vi "SendHardwareErrorStatus.vi"(8 "error in (no error)":errorcluster, 9 "EDP Hardware Labview Error Status":T1, 11 "Handle In":u32 format="%x") -> (0 "error out":errorcluster, 3 "Handle Out":u32 format="%x")   [LabVIEW 2020]
uses:
  <userlib>/Beckhoff-LabVIEW-Interface/_DependsOn/With TypeResolving/Write Sync Single TypeResolved.vi
panel:
  out "Has Matched? 3":bool
  out "Write Status 3":bool
  in  "WriteGrpSymbols 2":string[](array[string])=["192.168.0.20.1.1:851::GVL_LabviewDataShare.in_bAardvarkBoardError_labview", "192.168.0.20.1.1:851::GVL_LabviewDataShare.in_bAsic1CalibrationCompleted_labview", "192.168.0.20.1.1:851::GVL_LabviewDataShare.in_bAsic1CalibrationInProgress_labview", "192.168.0.20.1.1:851::GVL_LabviewDataShare.in_bAsic1CalibrationSuccess_labview", "192.168.0.20.1.1:851::GVL_LabviewDataShare.in_bAsic1FFTCompleted_labview", "192.168.0.20.1.1:851::GVL_LabviewDataShare.in_bAsic1FFTInProgress_labview", "192.168.0.20.1.1:851::GVL_LabviewDataShare.in_bAsic1FFTSuccess_labview", "192.168.0.20.1.1:851::GVL_LabviewDataShare.in_bAsic2CalibrationCompleted_labview", "192.168.0.20.1.1:851::GVL_LabviewDataShare.in_bAsic2CalibrationInProgress_labview", "192.168.0.20.1.1:851::GVL_LabviewDataShare.in_bAsic2CalibrationSuccess_labview", "192.168.0.20.1.1:851::GVL_LabviewDataShare.in_bAsic2FFTCompleted_labview", "192.168.0.20.1.1:851::GVL_LabviewDataShare.in_bAsic2FFTInProgress_labview", "192.168.0.20.1.1:851::GVL_LabviewDataShare.in_bAsic2FFTSuccess_labview", "192.168.0.20.1.1:851::GVL_LabviewDataShare.in_bCalResultsDBStoreSuccess_labview", "192.168.0.20.1.1:851::GVL_LabviewDataShare.in_bFFTResultsDBStoreSuccess_labview", "192.168.0.20.1.1:851::GVL_LabviewDataShare.in_bLabviewHandshakeBit", "192.168.0.20.1.1:851::GVL_LabviewDataShare.in_bLabviewResetComplete_labview", "192.168.0.20.1.1:851::GVL_LabviewDataShare.in_bLabviewResetSuccess_labview", "192.168.0.20.1.1:851::GVL_LabviewDataShare.in_bNIDaqError_labview", "192.168.0.20.1.1:851::GVL_LabviewDataShare.in_bPTC04BoardError_labview", "192.168.0.20.1.1:851::GVL_LabviewDataShare.in_bStartupInitializationCompleted_labview", "192.168.0.20.1.1:851::GVL_LabviewDataShare.in_bStartupInitializationSuccess_labview", "192.168.0.20.1.1:851::GVL_LabviewDataShare.in_strAsic1SerialNo_labview", "192.168.0.20.1.1:851::GVL_LabviewDataShare.in_strAsic2SerialNo_labview"]
  out "Write Status 2":bool
  out "Has Matched? 2":bool
  out "Write Status":bool
  out "Has Matched?":bool
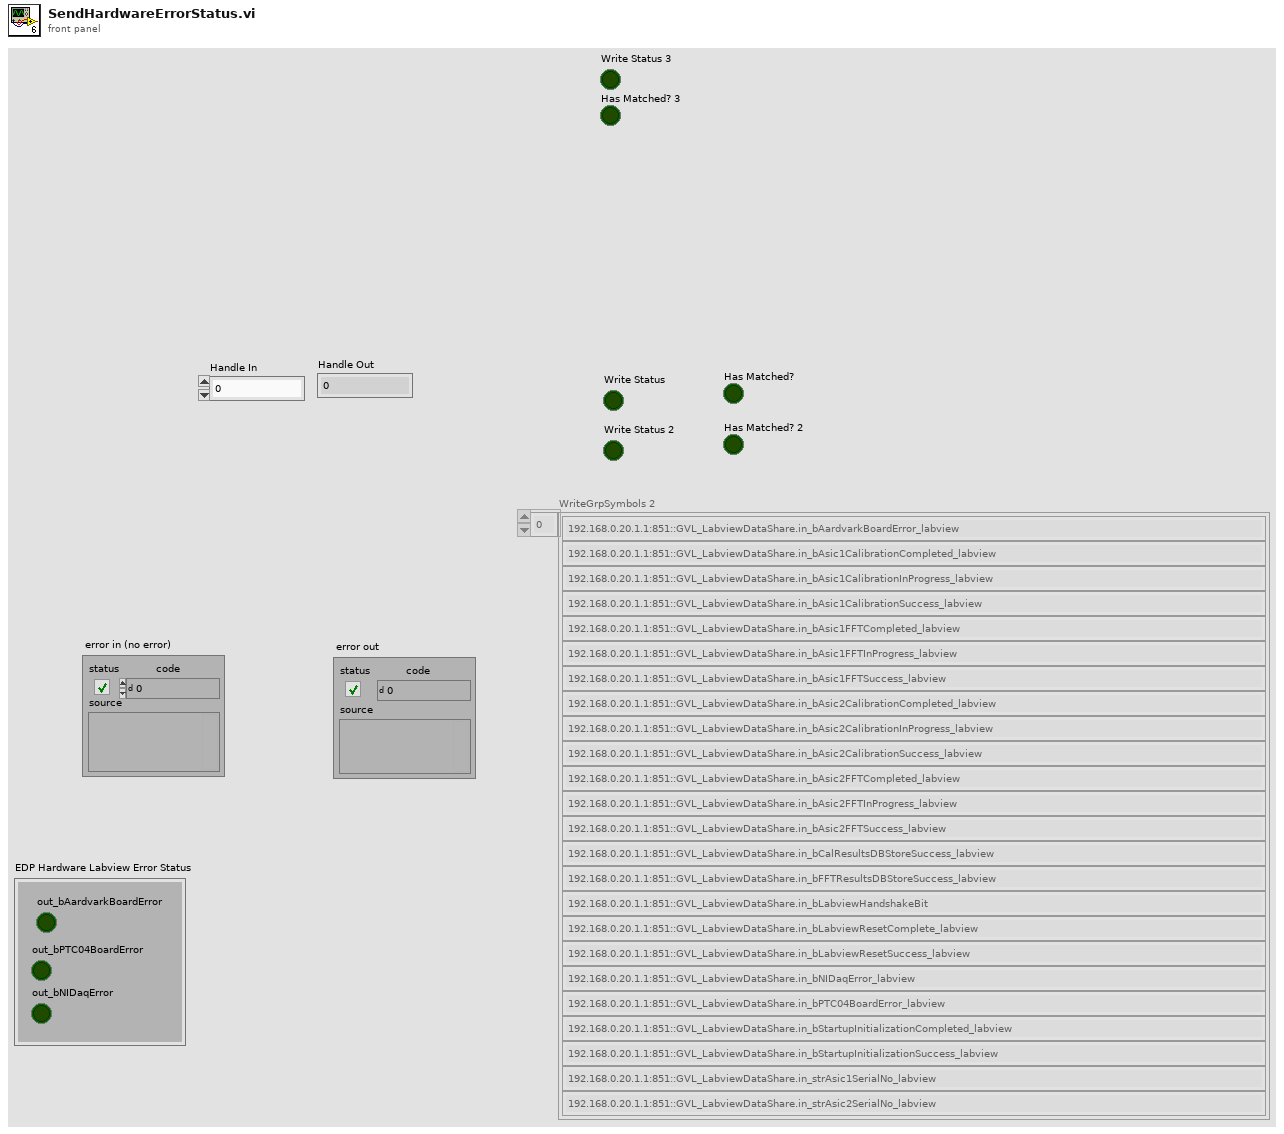
[diagram p1: front panel]
types:
  T1 = cluster{"out_bAardvarkBoardError":bool, "out_bPTC04BoardError":bool, "out_bNIDaqError":bool}
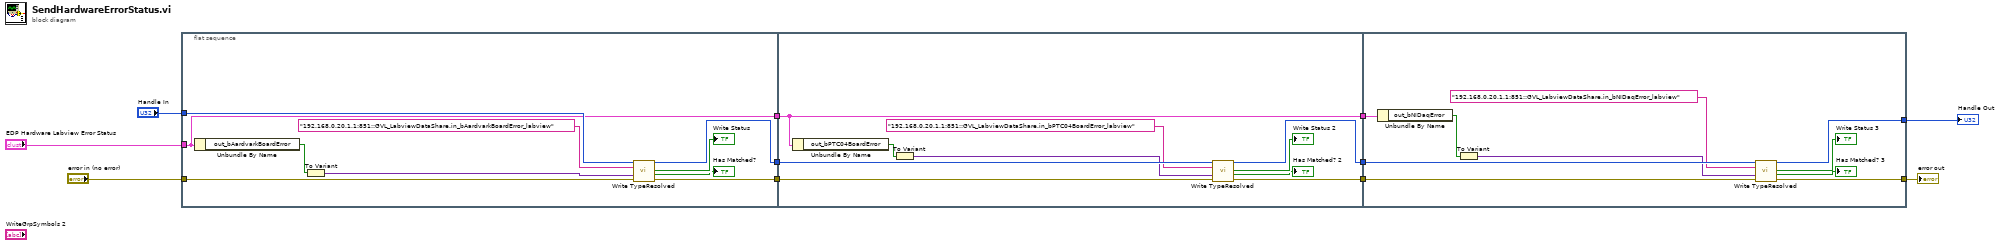
[diagram p0: block diagram]
diagram:
  n1 = flat-sequence {
    tunnel: "Handle In" -> [w21]
    tunnel: [w20] -> w11
    tunnel: [w19] -> w10
    tunnel: "error in (no error)" -> [w18]
    tunnel: "EDP Hardware Labview Error Status" -> [w15]
    tunnel: [w15] -> w9
    tunnel: w11 -> [w31]
    tunnel: w10 -> [w30]
    tunnel: w9 -> [w22]
    tunnel: [w24] -> w3
    tunnel: [w23] -> w2
    tunnel: [w22] -> w1
    tunnel: [w36] -> w5
    tunnel: [w38] -> w6
    tunnel: w3 -> [w39]
    tunnel: w2 -> [w37]
    tunnel: w1 -> [w41]
    frame #0 {
      n2 = Unbundle By Name(w15) -> ("out_bAardvarkBoardError"=w17:bool)
      n3 = To Variant(anything=w17) -> (Variant=w16:variant)
      n4 = call-poly <userlib>:"Write TypeResolved.vi"("Handle"=w21, "SymbolName"="192.168.0.20.1.1:851::GVL_LabviewDataShare.in_bAardvarkBoardError_labview", "WData"=w16, "error constant"=w18) -> ("Handle"=w20:u32, "Write Status?"=→"Write Status":bool, "Has Matched?"=→"Has Matched?":bool, "error out"=w19:errorcluster)  [unwired: 8 in]
    }
    frame #1 {
      n5 = Unbundle By Name(w22) -> ("out_bPTC04BoardError"=w29:bool)
      n6 = To Variant(anything=w29) -> (Variant=w28:variant)
      n7 = call-poly <userlib>:"Write TypeResolved.vi"("Handle"=w31, "SymbolName"="192.168.0.20.1.1:851::GVL_LabviewDataShare.in_bPTC04BoardError_labview", "WData"=w28, "error constant"=w30) -> ("Handle"=w23:u32, "Write Status?"=→"Write Status 2":bool, "Has Matched?"=→"Has Matched? 2":bool, "error out"=w24:errorcluster)  [unwired: 8 in]
    }
    frame #2 {
      n8 = Unbundle By Name(w41) -> ("out_bNIDaqError"=w40:bool)
      n9 = To Variant(anything=w40) -> (Variant=w34:variant)
      n10 = call-poly <userlib>:"Write TypeResolved.vi"("Handle"=w37, "SymbolName"="192.168.0.20.1.1:851::GVL_LabviewDataShare.in_bNIDaqError_labview", "WData"=w34, "error constant"=w39) -> ("Handle"=w36:u32, "Write Status?"=→"Write Status 3":bool, "Has Matched?"=→"Has Matched? 3":bool, "error out"=w38:errorcluster)  [unwired: 8 in]
    }
  }
  "error out" <- w6
  "Handle Out" <- w5
